vi "Read Async Scaled Data.vi"(5 "Component ID":u8, 7 "FPGA Interface":refnum<class "FPGA Interface.lvclass">, 8 "error in (no error)":errorcluster, 10 "Async Message":refnum<class "Async Message.lvclass">, 11 "Bus Controller in":refnum<class "Bus Controller.lvclass">) -> (0 "error out":errorcluster, 1 "Parameter Data":dbl[](array[numeric]), 2 "Parameters":string[](array[string]), 3 "Bus Controller out":refnum<class "Bus Controller.lvclass">)   [LabVIEW 2020, in "BCI-1553 API.lvlib" / "Bus Controller.lvclass"]
doc: "Reads scaled parameter data associated with the argument Asynchronous Message. An Asynchronous Message must be sent before this method will return valid data."
uses:
  Bus Controller.lvclass
  Frames & Messages/Async Message/Async Message.lvclass
  Dependencies/FPGA Interface/FPGA Interface.lvclass
  Bus Controller.lvclass/Bus Controller.ctl
  BCI-1553 API.lvlib
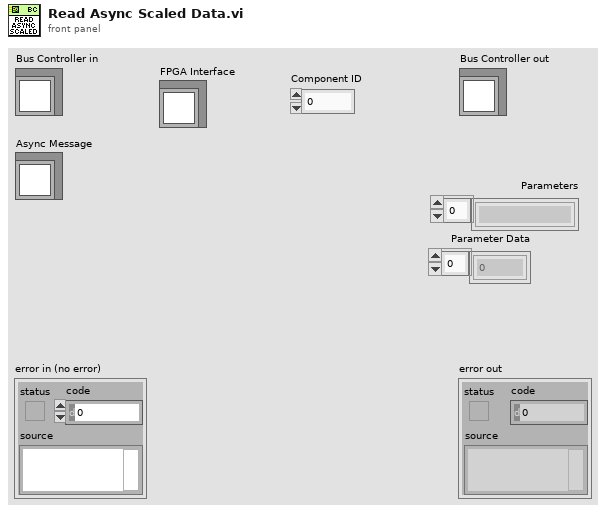
[diagram p1: front panel]
types:
  T1 = typedef "BCI-1553 API.lvlib/Async Message Pointers.ctl" = cluster{"HP Async Control Addresses":u16[], "HP Async Data Addresses":u16[], "LP Async Control Addresses":u16[], "LP Async Data Addresses":u16[]}
  T2 = typedef "BCI-1553 API.lvlib/Async Payload.ctl" = cluster{"Configuration Address":u16, "Configuration":u16[], "Data Address":u16, "Data":u16[], "Trigger Command":u16, "Command Type":enum16{"Transmit", "Receive"}}
  T3 = typedef "BCI-1553 API.lvlib/Scaling Information.ctl" = cluster{"Bit Offset":i32, "Bit Count":i32, "LSB Resolution":dbl, "2's Complement":bool, "Big Endian":bool, "Sign Bit":bool}
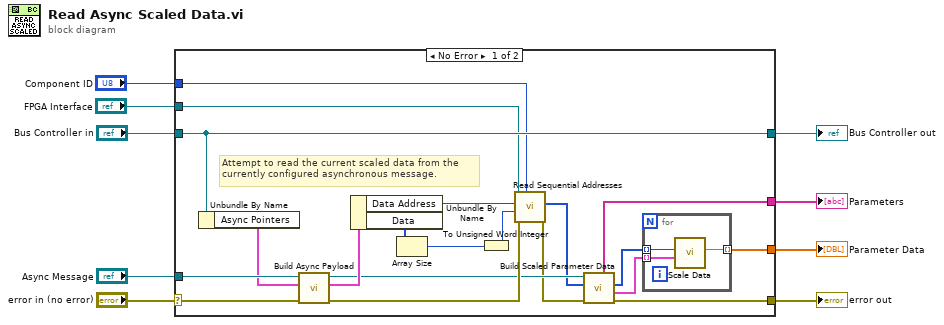
[diagram p0: block diagram]
diagram:
  n1 = case shown="No Error" "error in (no error)" {
    selector: "error in (no error)" -> [w27 w34]
    tunnel: [w15 w34] -> w7
    tunnel: [w26 w33] -> w6
    tunnel: "Bus Controller in" -> [w26 w33]
    tunnel: "Async Message" -> [w29 _]
    tunnel: "FPGA Interface" -> [w24 _]
    tunnel: "Component ID" -> [w23 _]
    tunnel: [w14 _] -> w2
    tunnel: [w11 _] -> w1
    frame No Error {
      # "Attempt to read the current scaled data from the\ncurrently configured asynchronous message."
      n2 = Unbundle By Name(w26) -> ("Async Pointers"=w28:T1)
      n3 = call-dynamic "Build Async Payload.vi"("error in (no error)"=w27, "Async Pointers"=w28, "Async Message in"=w29) -> ("error out"=w21:errorcluster, "Async Payload"=w25:T2, "Async Message out"=w18:refnum<class "Async Message.lvclass">)  [unwired: 6 in]
      n4 = Unbundle By Name(w25) -> ("Data Address"=w22:u16, "Data"=w20:u16[])
      n5 = Array Size(array=w20) -> (size(s)=w10:i32)
      n6 = To Unsigned Word Integer(number=w10) -> (unsigned 16bit integer=w19:u16)
      n7 = call-dynamic "Read Sequential Addresses.vi"("Target IC (1-8)"=w23, "error in (no error)"=w21, "Addresses to Read"=w19, "Starting Address"=w22, "FPGA Interface in"=w24) -> ("error out"=w16:errorcluster, "Data"=w17:u16[])  [unwired: 5 in]
      n8 = call-dynamic "Build Scaled Parameter Data.vi"("error in (no error)"=w16, "FPGA Data"=w17, "Async Message in"=w18) -> ("error out"=w15:errorcluster, "Parameter Scaling"=w12:T3[], "Parameter Raw Data"=w13:u64[], "Parameters"=w14:string[])  [unwired: 4 in, 1 out]
      n9 = for {
        tunnel: w12 -> [w32] mode=indexing
        tunnel: w13 -> [w31] mode=indexing
        tunnel: [w30] -> w11 mode=indexing
        n10 = call "Scale Data.vi"("Scaling Info"=w32, "Raw Value"=w31) -> ("Scaled Value"=w30:dbl)  [unwired: 8 in, 1 out]
      }
    }
    frame Error {
    }
  }
  "error out" <- w7
  "Bus Controller out" <- w6
  "Parameters" <- w2
  "Parameter Data" <- w1
